vi "Handle Incoming Packets.vi"(8 "error in (no error)":errorcluster, 10 "Incoming Packets":u8[](array[numeric]) format="%08b", 11 "ControlPacket in":refnum<class "ControlPacket.lvclass">) -> (0 "error out":errorcluster, 1 "Complete?":bool=TRUE, 2 "Remaining Packets":u8[](array[numeric]) format="%08b", 3 "ControlPacket out":refnum<class "ControlPacket.lvclass">)   [LabVIEW 2013, in "MQTT_Control_Packets.lvlib" / "ControlPacket.lvclass"]
uses:
  ControlPacket.lvclass
  ControlPacket.lvclass/ControlPacket.ctl
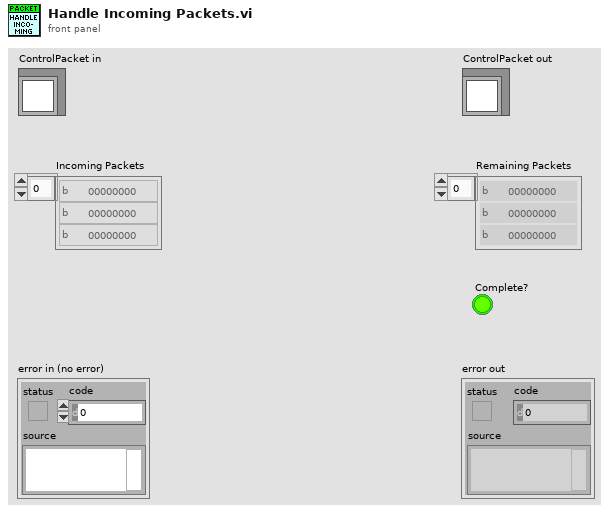
[diagram p1: front panel]
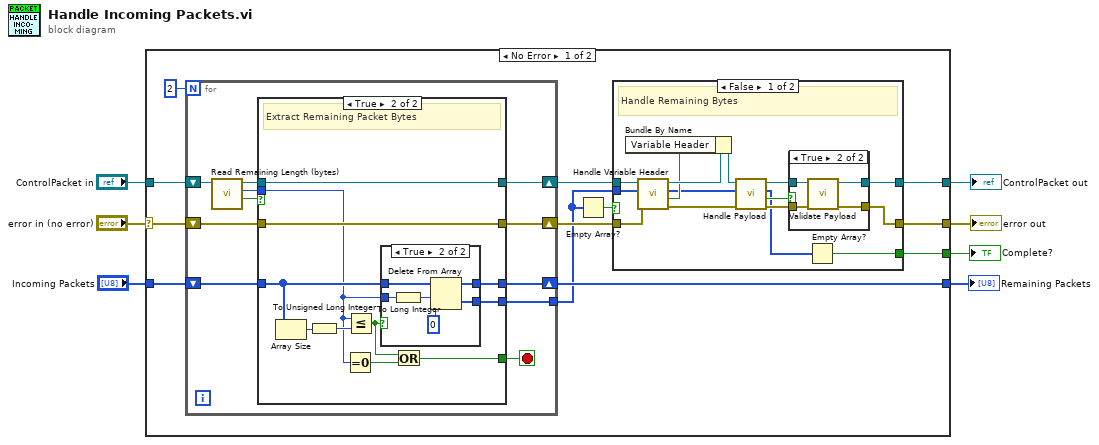
[diagram p0: block diagram]
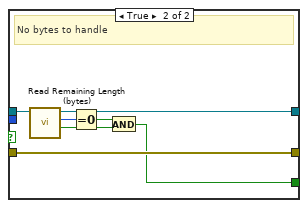
[diagram p3: hidden frame]
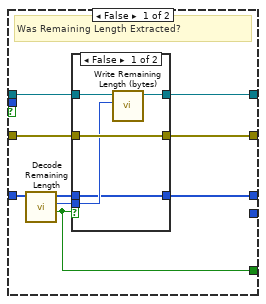
[diagram p4: hidden frame]
diagram:
  n1 = case shown="No Error" "error in (no error)" {
    selector: "error in (no error)" -> [w17 w96]
    tunnel: [w16 w96] -> w6
    tunnel: [w15 w95] -> w4
    tunnel: "ControlPacket in" -> [w19 w95]
    tunnel: "Incoming Packets" -> [w18 w94]
    tunnel: [w14 w94] -> w2
    tunnel: [w13 _] -> w1
    frame No Error {
      n2 = for {
        N: 2 -> [_]
        shift-right: [w57] -> w14
        shift-left: w18 -> [w58]
        shift-right: [w54] -> w9
        shift-left: w17 -> [w55]
        shift-right: [w56] -> w10
        shift-left: w19 -> [w53]
        tunnel: [w48] -> w8
        stop <- w49 stop-if-true
        n3 = call "Read Remaining Length (bytes).vi"("ControlPacket in"=w53) -> ("Length"=w51:bool, "Remaining Length (bytes)"=w50:u32, "ControlPacket out"=w52:refnum<class "ControlPacket.lvclass">)  [unwired: 8 in]
        n4 = case shown="True" w51 {
          tunnel: w58 -> [w67 w82]
          tunnel: [w66 w81] -> w57
          tunnel: [w63 w86] -> w56
          tunnel: w55 -> [w62 w85]
          tunnel: [w61 w85] -> w54
          tunnel: w52 -> [w60 w86]
          tunnel: w50 -> [_ w79]
          tunnel: [_ w80] -> w48
          tunnel: [w59 w76] -> w49
          frame False {
            # "Was Remaining Length Extracted?"
            n5 = call "Decode Remaining Length.vi"("Packet w/o 1st byte"=w67) -> ("Malformed Remaining Length"=w59:bool, "Remaining Length (bytes)"=w64:u32, "Remaining Packet"=w65:u8[])  [unwired: 8 in]
            n6 = case shown="False" w59 {
              tunnel: [w68 w75] -> w66
              tunnel: w65 -> [w68 w75]
              tunnel: w64 -> [w69 _]
              tunnel: [w71 w74] -> w63
              tunnel: w60 -> [w72 w74]
              tunnel: w62 -> [w70 w73]
              tunnel: [w70 w73] -> w61
              frame False {
                n7 = call "Write Remaining Length (bytes).vi"("Remaining Length (bytes)"=w69, "ControlPacket in"=w72) -> ("ControlPacket out"=w71:refnum<class "ControlPacket.lvclass">)  [unwired: 9 in]
              }
              frame True {
              }
            }
          }
          frame True {
            # "Extract Remaining Packet Bytes"
            n8 = Array Size(array=w82) -> (size(s)=w84:i32)
            n9 = To Unsigned Long Integer(number=w84) -> (unsigned 32bit integer=w83:u32)
            n10 = Equal To 0?(x=w79) -> (x = 0?=w77:bool)
            n11 = Less Or Equal?(x=w79, y=w83) -> (x <= y?=w78:bool)
            n12 = case shown="True" w78 {
              tunnel: w82 -> [w87 w93]
              tunnel: w79 -> [_ w92]
              tunnel: [_ w90] -> w80
              tunnel: [w87 w89] -> w81
              frame False {
              }
              frame True {
                n13 = To Long Integer(number=w92) -> (32bit integer=w88:i32)
                n14 = Delete From Array(array=w93, length=w88, index=0) -> (deleted portion=w90:u8[], array with subset deleted=w89:u8[])
              }
            }
            n15 = Or(x=w78, y=w77) -> (x .or. y?=w76:bool)
          }
        }
      }
      n16 = Empty Array?(array=w8) -> (empty?=w11:bool)
      n17 = case shown="False" w11 {
        tunnel: w10 -> [w33 w42]
        tunnel: [w25 w41] -> w15
        tunnel: w9 -> [w32 w47]
        tunnel: [w23 w47] -> w16
        tunnel: w8 -> [w34 _]
        tunnel: [w20 w43] -> w13
        frame False {
          # "Handle Remaining Bytes"
          n18 = call-dynamic "Handle Variable Header.vi"("error in (no error)"=w32, "Incoming Packets"=w34, "ControlPacket in"=w33) -> ("error out"=w27:errorcluster, "Variable Header Complete?"=w30:bool, "Remaining Packets"=w28:u8[], "ControlPacket out"=w31:refnum<class "ControlPacket.lvclass">)  [unwired: 5 in]
          n19 = Bundle By Name(cluster=w31, "Variable Header"=w30) -> (w29:refnum<class "ControlPacket.lvclass">)
          n20 = call "Handle Payload.vi"("error in (no error)"=w27, "Incoming Packets"=w28, "ControlPacket in"=w29) -> ("error out"=w24:errorcluster, "Payload Complete?"=w22:bool, "Remaining Packets"=w21:u8[], "ControlPacket out"=w26:refnum<class "ControlPacket.lvclass">)  [unwired: 5 in]
          n21 = case shown="True" w22 {
            tunnel: w26 -> [w36 w40]
            tunnel: [w36 w39] -> w25
            tunnel: w24 -> [w35 w38]
            tunnel: [w35 w37] -> w23
            frame False {
            }
            frame True {
              n22 = call-dynamic "Validate Payload.vi"("error in (no error)"=w38, "ControlPacket in"=w40) -> ("error out"=w37:errorcluster, "ControlPacket out"=w39:refnum<class "ControlPacket.lvclass">)  [unwired: 7 in, 1 out]
            }
          }
          n23 = Empty Array?(array=w21) -> (empty?=w20:bool)
        }
        frame True {
          # "No bytes to handle"
          n24 = call "Read Remaining Length (bytes).vi"("ControlPacket in"=w42) -> ("Length"=w44:bool, "Remaining Length (bytes)"=w46:u32, "ControlPacket out"=w41:refnum<class "ControlPacket.lvclass">)  [unwired: 8 in]
          n25 = Equal To 0?(x=w46) -> (x = 0?=w45:bool)
          n26 = And(x=w45, y=w44) -> (x .and. y?=w43:bool)
        }
      }
    }
    frame Error {
    }
  }
  "error out" <- w6
  "ControlPacket out" <- w4
  "Remaining Packets" <- w2
  "Complete?" <- w1
